vi "Text Label Test.vi"() -> ()   [LabVIEW 2015]
uses:
  D:/Experiment VIs/Utility VIs/Math VIs/LinSpace (x0-dx-npts).vi
panel:
  in  "Slide":dbl(slide) caption="Time" min=0.0 scale=0.0..12.0
  out "XY Graph":cluster{"Freq":dbl[], "Threshold":dbl[]}[](graph)
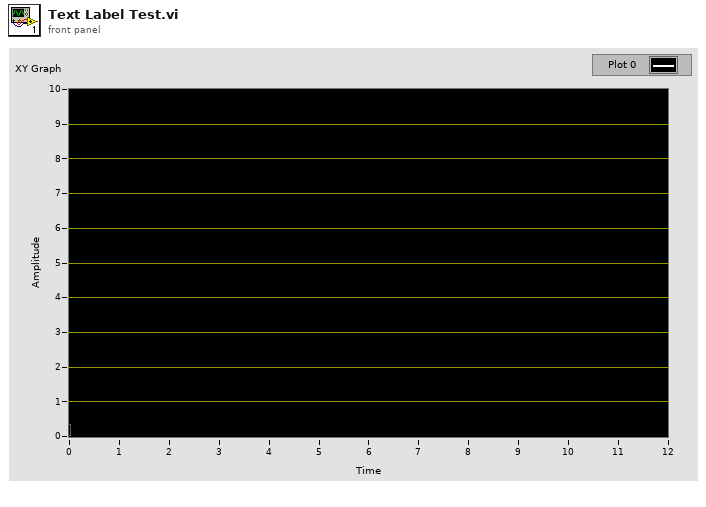
[diagram p1: front panel]
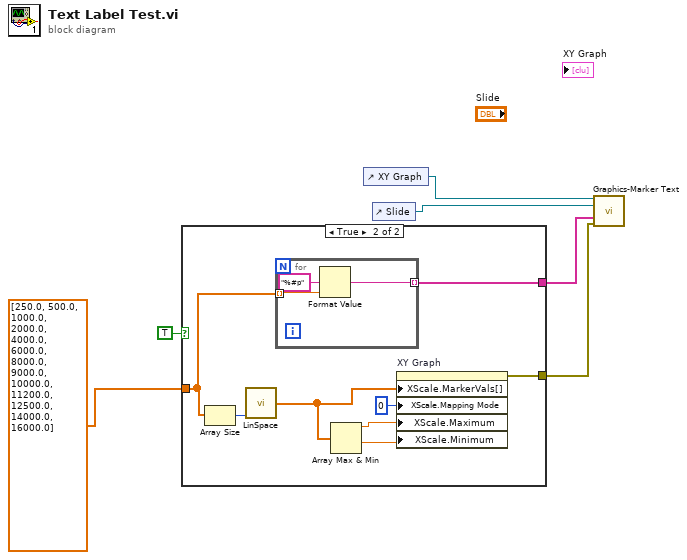
[diagram p0: block diagram]
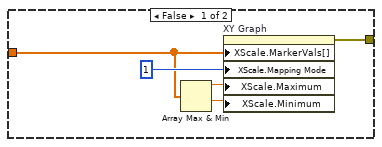
[diagram p2: hidden frame]
diagram:
  n1 = case shown="True" TRUE {
    tunnel: [w11 w19] -> w5
    tunnel: dbl[] [250.0, 500.0, 1000.0, 2000.0, 4000.0, 6000.0, 8000.0, 9000.0, 10000.0, 11200.0, 12500.0, 14000.0, 16000.0] ("X Scale.Marker Values[]") -> [w7 w13]
    tunnel: [_ w12] -> w1
    frame False {
      n2 = Array Max & Min(array=w7) -> (max value=w9:dbl, min value=w8:dbl)  [unwired: 2 out]
      n3 = property on="XY Graph" class="XYGraph (strict)"("XScale.MarkerVals[]"=w7, "XScale.Mapping Mode"=u8 1 ("X Scale.Mapping Mode"), "XScale.Maximum"=w9, "XScale.Minimum"=w8) -> (error out=w11:errorcluster)  [unwired: 2 in, 1 out]
    }
    frame True {
      n4 = Array Size(array=w13) -> (size(s)=w15:i32)
      n5 = call-poly "LinSpace.vi"("npts"=w15) -> ("Array"=w14:dbl[])  [unwired: 3 in, 1 out]
      n6 = for {
        tunnel: w13 -> [w22] mode=indexing
        tunnel: [w20] -> w12 mode=indexing
        n7 = Format Value(format string="%#p", value (0)=w22) -> (output string=w20:string)  [unwired: 1 in]
      }
      n8 = Array Max & Min(array=w14) -> (max value=w17:dbl, min value=w16:dbl)  [unwired: 2 out]
      n9 = property on="XY Graph" class="XYGraph (strict)"("XScale.MarkerVals[]"=w14, "XScale.Mapping Mode"=u8 0 ("X Scale.Mapping Mode"), "XScale.Maximum"=w17, "XScale.Minimum"=w16) -> (error out=w19:errorcluster)  [unwired: 2 in, 1 out]
    }
  }
  n10 = control-ref of="XY Graph"() -> (w3:refnum<vi>)
  n11 = control-ref of="Slide"() -> (w6:refnum<vi>)
  n12 = call "Graphics-Marker Text.vi"("XYGraph"=w3, "Slider"=w6, "Text Labels[]"=w1, "error in (no error)"=w5) -> ()  [unwired: 11 in, 1 out]
